vi "Monitors_EPR_v03.vi"(0 "IIR filter specifications":T1={"Topology"=enum."Butterworth", "Type"=enum."Lowpass", "Order"=1, "Lower Fc"=100.0, "Upper Fc"=200.0, "PB Ripple"=1.0, "SB Attenuation"=60.0} {"PB Ripple" format="%0.2f"; "SB Attenuation" format="%0.2f"; "Lower Fc" format="%0.2p"; "Upper Fc" format="%0.2p"}, 2 "reset SN":bool, 5 "Shot noise start":bool, 6 "wfm":waveform(dbl)[](array[waveform]), 10 "hbar":dbl, 16 "Wait(mSec)":u32 caption="Count(mSec)") -> (11 "Var(p1+p3)":dbl format="%0.2f", 13 "Var(p2+p3)":dbl format="%0.2f", 15 "Var(p1+p2)":dbl format="%0.2f", 17 "conditional variance B1|A":dbl, 20 "covariance B01":dbl, 21 "Var(x1-x2)":dbl format="%0.2f", 22 "covariance B0A":dbl, 23 "covariance B1A":dbl, 24 "Var(x2-x3)":dbl format="%0.2f", 25 "conditional variance B0|1":dbl, 26 "conditional variance B0|A":dbl, 27 "Var(x1-x3)":dbl format="%0.2f")   [LabVIEW 2013]
uses:
  <vilib>/Analysis/5stat.llb/RMS (DBL).vi
  <vilib>/Analysis/baseanly.llb/Mean (DBL).vi
  shotnoise.vi
  <vilib>/measure/maspectr.llb/FFT Spectrum (Mag-Phase) for N Chan.vi
  <vilib>/measure/matone.llb/Extract Single Tone Information N Chan.vi
  <vilib>/measure/macond.llb/IIR Filter for N Chan.vi
  <vilib>/measure/NI_MAPro.lvlib
  <vilib>/Analysis/NI_AALPro.lvlib
  <vilib>/Analysis/NI_AALBase.lvlib
panel:
  out "Waveform Graph 2":cluster{"f0":dbl, "df":dbl, "magnitude":dbl[]}[](graph)
  out "detected frequencies":dbl[](array[numeric]) format="%.2p"
  out "ch12":dbl
  out "ch02":dbl
  out "ch01":dbl
  out "Waveform Graph":waveform(dbl)[](graph)
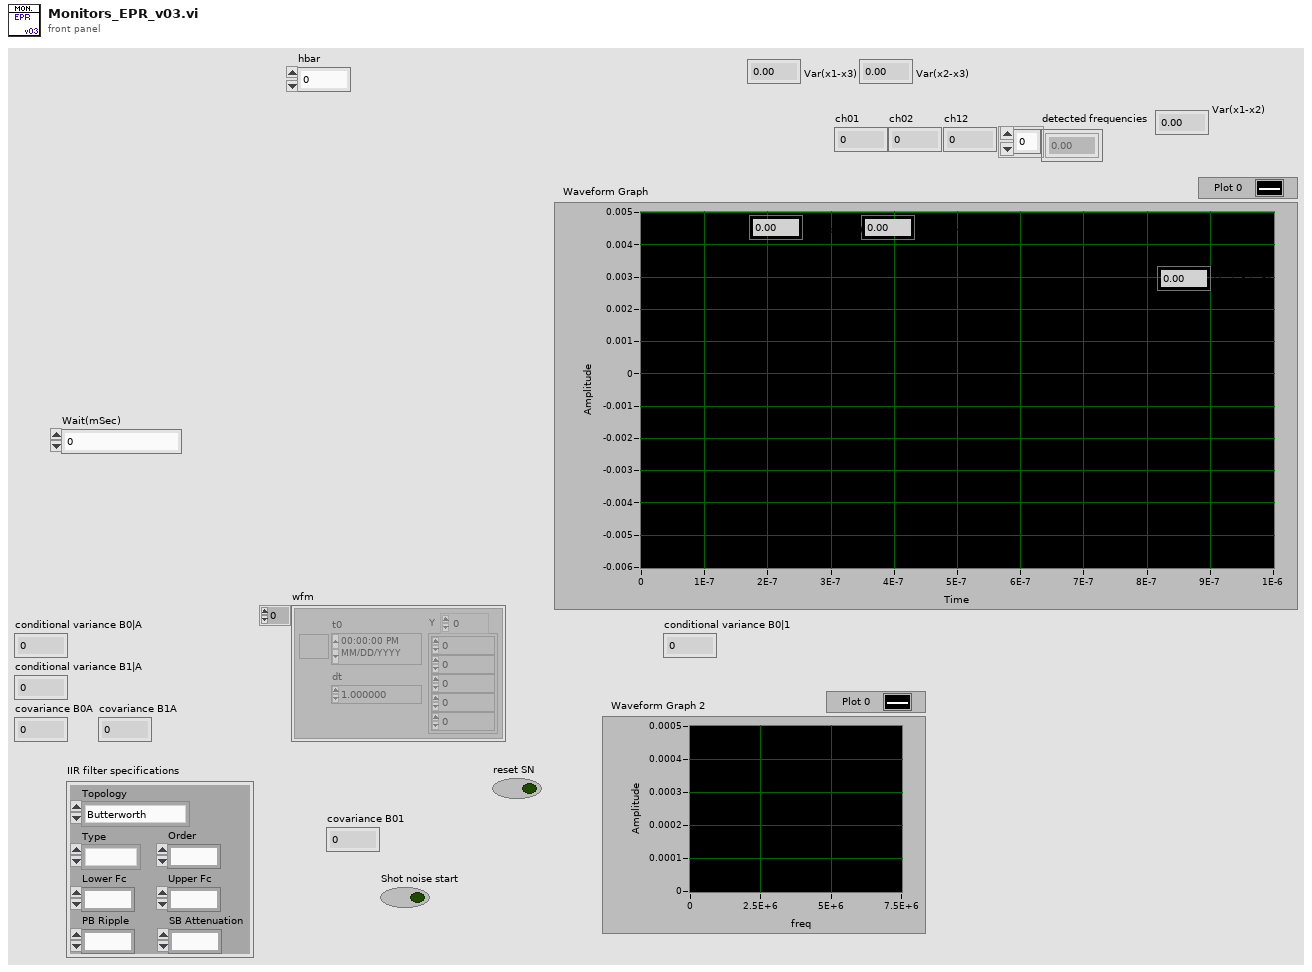
[diagram p1: front panel]
types:
  T1 = cluster{"Topology":enum16{"Off", "Butterworth", "Chebyshev", "Inverse Chebyshev", "Elliptic", "Bessel"}, "Type":enum16{"Lowpass", "Highpass", "Bandpass", "Bandstop"}, "Order":i32, "Lower Fc":dbl, "Upper Fc":dbl, "PB Ripple":dbl, "SB Attenuation":dbl}
  T2 = cluster{"approx freq. (optional)":dbl, "search (+/- % of Fsampl.)":dbl}
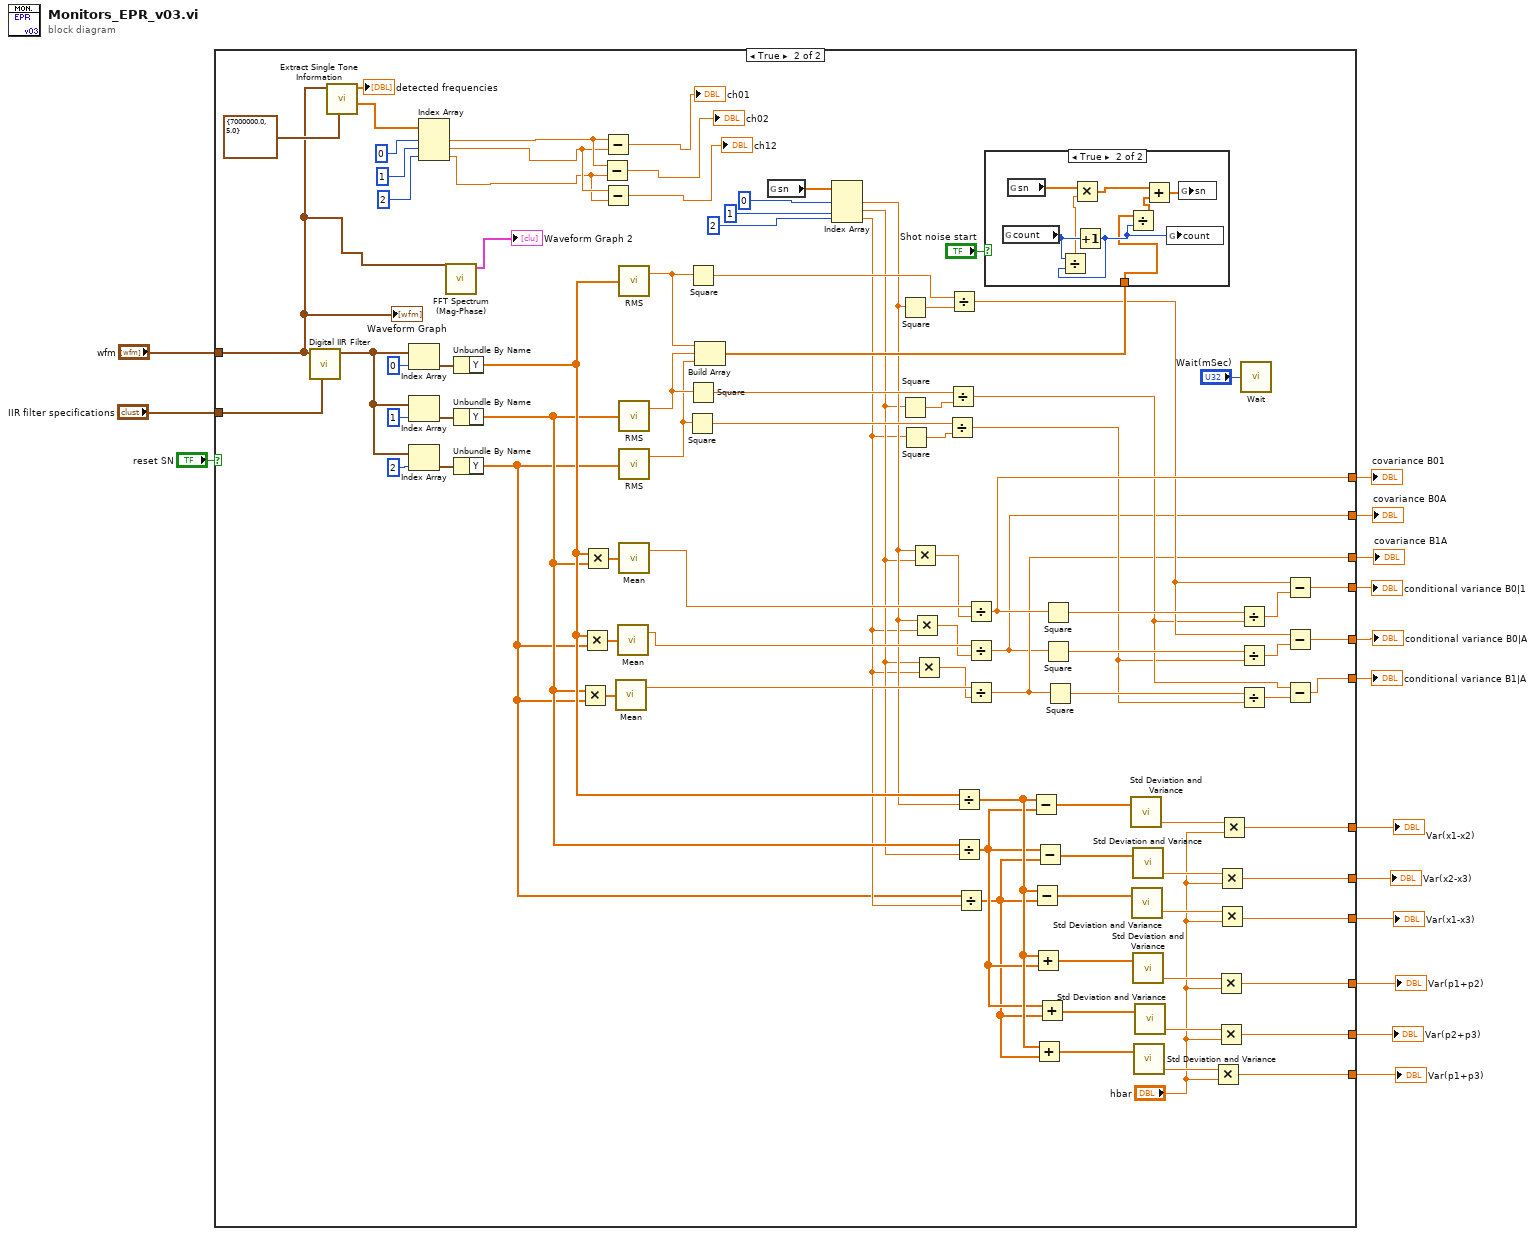
[diagram p0: block diagram]
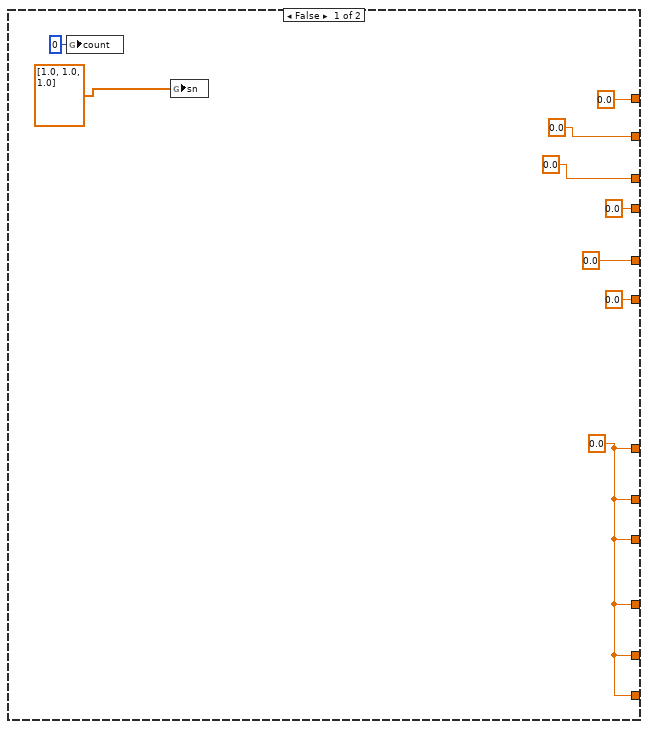
[diagram p2: hidden frame]
diagram:
  n1 = case shown="True" "reset SN" {
    tunnel: "IIR filter specifications" -> [_ w114]
    tunnel: "wfm" -> [_ w53]
    tunnel: [0.0 w94] -> w13
    tunnel: [0.0 w93] -> w11
    tunnel: [0.0 w79] -> w10
    tunnel: [0.0 w70] -> w9
    tunnel: [0.0 w67] -> w8
    tunnel: [0.0 w69] -> w7
    tunnel: [w16 w29] -> w6
    tunnel: [w16 w27] -> w5
    tunnel: [w16 w28] -> w4
    tunnel: [w16 w26] -> w1
    tunnel: [w16 w36] -> w2
    tunnel: [w16 w25] -> w3
    frame False {
      w16 = 0.0 ("variance")
      n2 = global write "shotnoise.vi" "count"(i64 0 ("count")) -> ()
      n3 = global write "shotnoise.vi" "sn"(dbl[] [1.0, 1.0, 1.0] ("sn")) -> ()
    }
    frame True {
      n4 = call-poly <vilib>:"Digital IIR Filter.vi"("IIR filter specifications"=w114, "signal(s) in"=w53) -> ("signal(s) out"=w91:waveform(dbl)[])  [unwired: 4 in, 5 out]
      n5 = call-poly <vilib>:"Extract Single Tone Information.vi"("advanced search"=T2 {"approx freq. (optional)"=7000000.0, "search (+/- % of Fsampl.)"=5.0}, "time signals in"=w53) -> ("detected phases (deg)"=w63:dbl[], "detected frequencies"=→"detected frequencies":dbl[])  [unwired: 4 in, 4 out]
      n6 = Index Array(array=w91, index=0) -> (element=w97:waveform(dbl))
      n7 = Index Array(array=w91, index=1) -> (element=w100:waveform(dbl))
      n8 = Index Array(array=w91, index=2) -> (element=w90:waveform(dbl))
      n9 = Index Array(array=w63, index #1=0 ("index"), index #2=1 ("index"), index #3=2 ("index")) -> (element #1=w62:dbl, element #2=w61:dbl, element #3=w60:dbl)
      n10 = call-poly <vilib>:"FFT Spectrum (Mag-Phase).vi"("time signals"=w53) -> ("magnitudes"=→"Waveform Graph 2":cluster{"f0":dbl, "df":dbl, "magnitude":dbl[]}[])  [unwired: 6 in, 4 out]
      n11 = Unbundle By Name(w97) -> ("Y"=w52:dbl[])
      n12 = Unbundle By Name(w100) -> ("Y"=w50:dbl[])
      n13 = Unbundle By Name(w90) -> ("Y"=w47:dbl[])
      n14 = Multiply(x=w50, y=w47) -> (x*y=w77:dbl[])
      n15 = Multiply(x=w52, y=w47) -> (x*y=w89:dbl[])
      n16 = Multiply(x=w52, y=w50) -> (x*y=w112:dbl[])
      n17 = Subtract(x=w62, y=w60) -> (x-y=→"ch02":dbl)
      n18 = Subtract(x=w62, y=w61) -> (x-y=→"ch01":dbl)
      n19 = Subtract(x=w61, y=w60) -> (x-y=→"ch12":dbl)
      n20 = call-poly <vilib>:"Mean.vi"("X"=w77) -> ("mean"=w76:dbl)  [unwired: 1 out]
      n21 = call-poly <vilib>:"Mean.vi"("X"=w89) -> ("mean"=w83:dbl)  [unwired: 1 out]
      n22 = call-poly <vilib>:"RMS.vi"("X"=w52) -> ("rms value"=w108:dbl)  [unwired: 1 out]
      n23 = call-poly <vilib>:"RMS.vi"("X"=w50) -> ("rms value"=w110:dbl)  [unwired: 1 out]
      n24 = call-poly <vilib>:"RMS.vi"("X"=w47) -> ("rms value"=w86:dbl)  [unwired: 1 out]
      n25 = call-poly <vilib>:"Mean.vi"("X"=w112) -> ("mean"=w113:dbl)  [unwired: 1 out]
      n26 = Square(x=w86) -> (x^2=w85:dbl)
      n27 = Square(x=w108) -> (x^2=w109:dbl)
      n28 = Square(x=w110) -> (x^2=w111:dbl)
      n29 = Build Array(w108, w110, w86) -> (w107:dbl[])
      n30 = global read "shotnoise.vi" "sn"() -> (w99:dbl[])
      n31 = Index Array(array=w99, index #1=0 ("index"), index #2=1 ("index"), index #3=2 ("index")) -> (element #1=w51:dbl, element #2=w49:dbl, element #3=w48:dbl)
      n32 = Square(x=w51) -> (x^2=w104:dbl)
      n33 = Square(x=w49) -> (x^2=w105:dbl)
      n34 = Square(x=w48) -> (x^2=w84:dbl)
      n35 = Multiply(x=w51, y=w49) -> (x*y=w106:dbl)
      n36 = Multiply(x=w51, y=w48) -> (x*y=w82:dbl)
      n37 = Multiply(x=w49, y=w48) -> (x*y=w75:dbl)
      n38 = Divide(x=w85, y=w84) -> (x/y=w71:dbl)
      n39 = Divide(x=w111, y=w105) -> (x/y=w72:dbl)
      n40 = Divide(x=w109, y=w104) -> (x/y=w78:dbl)
      n41 = Divide(x=w52, y=w51) -> (x/y=w40:dbl[])
      n42 = Divide(x=w50, y=w49) -> (x/y=w39:dbl[])
      n43 = Divide(x=w47, y=w48) -> (x/y=w38:dbl[])
      n44 = Divide(x=w113, y=w106) -> (x/y=w93:dbl)
      n45 = Divide(x=w83, y=w82) -> (x/y=w67:dbl)
      n46 = Divide(x=w76, y=w75) -> (x/y=w69:dbl)
      n47 = case shown="True" "Shot noise start" {
        tunnel: w107 -> [_ w116]
        frame False {
        }
        frame True {
          n48 = global read "shotnoise.vi" "count"() -> (w121:i64)
          n49 = global read "shotnoise.vi" "sn"() -> (w120:dbl[])
          n50 = Increment(x=w121) -> (x+1=w117:i64)
          n51 = Divide(x=w121, y=w117) -> (x/y=w119:dbl)
          n52 = Multiply(x=w120, y=w119) -> (x*y=w118:dbl[])
          n53 = Divide(x=w116, y=w117) -> (x/y=w115:dbl[])
          n54 = Add(x=w118, y=w115) -> (x+y=w122:dbl[])
          n55 = global write "shotnoise.vi" "count"(w117) -> ()
          n56 = global write "shotnoise.vi" "sn"(w122) -> ()
        }
      }
      n57 = Subtract(x=w40, y=w39) -> (x-y=w46:dbl[])
      n58 = Subtract(x=w40, y=w38) -> (x-y=w45:dbl[])
      n59 = Add(x=w40, y=w39) -> (x+y=w41:dbl[])
      n60 = Add(x=w40, y=w38) -> (x+y=w42:dbl[])
      n61 = Subtract(x=w39, y=w38) -> (x-y=w44:dbl[])
      n62 = Add(x=w39, y=w38) -> (x+y=w43:dbl[])
      n63 = Square(x=w93) -> (x^2=w102:dbl)
      n64 = Square(x=w67) -> (x^2=w81:dbl)
      n65 = Square(x=w69) -> (x^2=w74:dbl)
      n66 = call <vilib>:"Std Deviation and Variance.vi"("X"=w46) -> ("variance"=w31:dbl)  [unwired: 1 in, 2 out]
      n67 = call <vilib>:"Std Deviation and Variance.vi"("X"=w45) -> ("variance"=w33:dbl)  [unwired: 1 in, 2 out]
      n68 = call <vilib>:"Std Deviation and Variance.vi"("X"=w44) -> ("variance"=w32:dbl)  [unwired: 1 in, 2 out]
      n69 = call <vilib>:"Std Deviation and Variance.vi"("X"=w41) -> ("variance"=w34:dbl)  [unwired: 1 in, 2 out]
      n70 = call <vilib>:"Std Deviation and Variance.vi"("X"=w42) -> ("variance"=w37:dbl)  [unwired: 1 in, 2 out]
      n71 = call <vilib>:"Std Deviation and Variance.vi"("X"=w43) -> ("variance"=w35:dbl)  [unwired: 1 in, 2 out]
      n72 = Multiply(x=w37, y="hbar") -> (x*y=w36:dbl)
      n73 = Multiply(x=w34, y="hbar") -> (x*y=w26:dbl)
      n74 = Multiply(x=w35, y="hbar") -> (x*y=w25:dbl)
      n75 = Multiply(x=w32, y="hbar") -> (x*y=w28:dbl)
      n76 = Multiply(x=w33, y="hbar") -> (x*y=w27:dbl)
      n77 = Multiply(x=w31, y="hbar") -> (x*y=w29:dbl)
      n78 = Divide(x=w102, y=w72) -> (x/y=w103:dbl)
      n79 = Divide(x=w81, y=w71) -> (x/y=w80:dbl)
      n80 = Divide(x=w74, y=w71) -> (x/y=w73:dbl)
      n81 = call "Wait"("Count(mSec)"="Wait(mSec)") -> ()  [unwired: 1 out]
      n82 = Subtract(x=w78, y=w103) -> (x-y=w94:dbl)
      n83 = Subtract(x=w78, y=w80) -> (x-y=w79:dbl)
      n84 = Subtract(x=w72, y=w73) -> (x-y=w70:dbl)
      "Waveform Graph" <- w53
    }
  }
  "conditional variance B0|1" <- w13
  "covariance B01" <- w11
  "conditional variance B0|A" <- w10
  "conditional variance B1|A" <- w9
  "covariance B0A" <- w8
  "covariance B1A" <- w7
  "Var(x1-x2)" <- w6
  "Var(x1-x3)" <- w5
  "Var(x2-x3)" <- w4
  "Var(p1+p2)" <- w1
  "Var(p1+p3)" <- w2
  "Var(p2+p3)" <- w3
